vi "Configure Debug Mode.vi"(8 "error in (no error)":errorcluster, 10 "Debug Mode? [F]":bool, 11 "Instrument in":refnum<class "Instrument.lvclass">) -> (0 "error out":errorcluster, 3 "Instrument out":refnum<class "Instrument.lvclass">)   [LabVIEW 2019, in "Instrument.lvlib" / "Instrument.lvclass"]
uses:
  Instrument.lvclass
  <userlib>/LevyLab/Debug/Attribute.Debug/DebugBehavior.ctl
  <userlib>/LevyLab/Debug/Attribute.Debug/Attribute.Debug.lvclass
  <userlib>/LevyLab/Debug/Debug.lvlib
  C:/Program Files (x86)/National Instruments/LabVIEW 2019/vi.lib/JKI/JKI SMO/SMO/SMO.lvclass
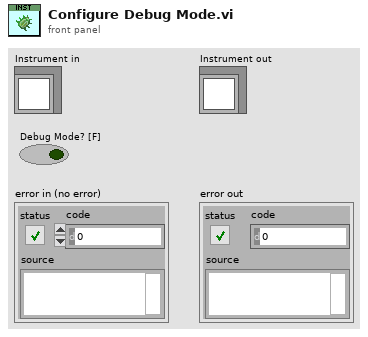
[diagram p1: front panel]
types:
  T1 = typedef "Debug.lvlib/Attribute.Debug.lvclass/DebugBehavior.ctl" = enum16{"Normal", "Debug"}
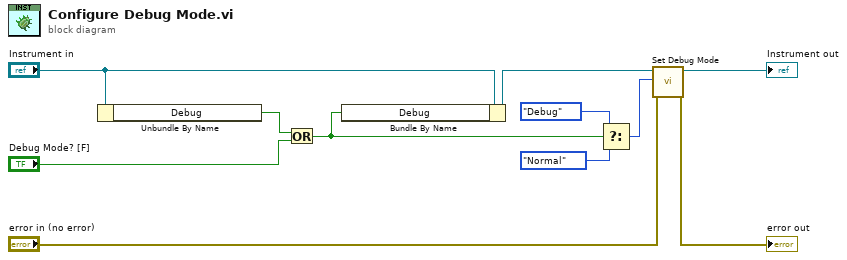
[diagram p0: block diagram]
diagram:
  n1 = Unbundle By Name("Instrument in") -> ("Debug"=w2:bool)
  n2 = Or(x=w2, y="Debug Mode? [F]") -> (x .or. y?=w11:bool)
  n3 = Bundle By Name(cluster="Instrument in", "Debug"=w11) -> (w10:refnum<class "Instrument.lvclass">)
  n4 = Select(t=DebugBehavior."Debug" ("Behavior"), s=w11, f=DebugBehavior."Normal" ("Behavior")) -> (s? t:f=w4:T1)
  n5 = call <userlib>:"Set Debug Mode.vi"("error in (no error)"="error in (no error)", "Behavior"=w4, "SMO"=w10) -> ("error out"=→"error out":errorcluster, "SMO out"=→"Instrument out":refnum<class "Instrument.lvclass">)  [unwired: 7 in]
